vi "niRFSTS Digitizer Initialize.vi"(8 "error in (no error)":errorcluster, 10 "Instrument Type Id":string, 11 "TSM Context":T1) -> (0 "error out":errorcluster)   [LabVIEW 2014]
uses:
  <vilib>/NI_TestStand_SemiconductorModule/NI_TestStand_Semiconductor_Module.lvlibp/PinMap/General/SemiconductorModuleContext.ctl
  <vilib>/NI_TestStand_SemiconductorModule/NI_TestStand_Semiconductor_Module.lvlibp
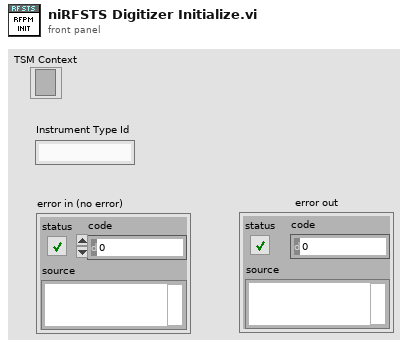
[diagram p1: front panel]
types:
  T1 = typedef "NI_TestStand_Semiconductor_Module.lvlibp/SemiconductorModuleContext.ctl" = refnum<k7>
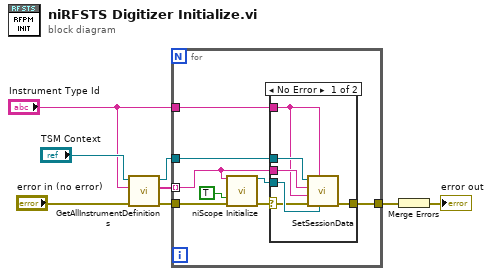
[diagram p0: block diagram]
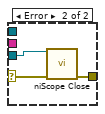
[diagram p2: hidden frame]
diagram:
  n1 = call <vilib>:"GetAllInstrumentDefinitions.vi"("error in (no error)"="error in (no error)", "Instrument Type Id"="Instrument Type Id", "Semiconductor Module Context"="TSM Context") -> ("error out"=w5:errorcluster, "Instrument Names"=w6:string[], "Semiconductor Module Context Out"=w7:T1)  [unwired: 4 in, 2 out]
  n2 = for {
    tunnel: [w16] -> w2
    tunnel: w5 -> [w13]
    tunnel: w6 -> [w14] mode=indexing
    tunnel: w7 -> [w15]
    tunnel: "Instrument Type Id" -> [w9]
    n3 = call <instrlib>:"niScope Initialize.vi"("resource name"=w14, "reset device"=TRUE ("Reset"), "error in"=w13) -> ("instrument handle"=w12:refnum<k15>, "error out"=w11:errorcluster)  [unwired: 11 in]
    n4 = case shown="No Error" w11 {
      selector: w11 -> [w19 w25]
      tunnel: [w17 w24] -> w16
      tunnel: w15 -> [w22 _]
      tunnel: w12 -> [w20 w23]
      tunnel: w14 -> [w21 _]
      tunnel: w9 -> [w18 _]
      frame No Error {
        n5 = call <vilib>:"SetSessionData.vi"("Session Data"=w20, "Instrument Type Id"=w18, "error in (no error)"=w19, "Channel Group Id"=w18, "Instrument Name"=w21, "Semiconductor Module Context"=w22) -> ("error out"=w17:errorcluster)  [unwired: 4 in, 1 out]
      }
      frame Error {
        n6 = call <instrlib>:"niScope Close.vi"("instrument handle"=w23, "error in"=w25) -> ("error out"=w24:errorcluster)  [unwired: 13 in]
      }
    }
  }
  n7 = Merge Errors(w2) -> (→"error out":errorcluster)
